vi "ENCOER_SUBVI.vi"(3 "Reset_Z":bool, 4 "Reset_Y":bool, 5 "Reset_X":bool) -> (0 "Position_Z":i16, 1 "Position_Y":i16, 2 "Position_X":i16)   [LabVIEW 2017]
uses:
  <vilib>/Platform/TimedLoop/XDataNode/timing_clust.ctl
  <vilib>/Platform/TimedLoop/XDataNode/nitl_modes.ctl
  <vilib>/Platform/TimedLoop/XDataNode/wakeup.ctl
  <vilib>/rvi/Emulation/niFpgaSctlEmulationGetInTimedLoop.vi
  <vilib>/rvi/Emulation/niFpgaEmulationReportErrorSimple.vi
  <vilib>/rvi/Emulation/niFpgaGetClockAttributes.vi
  <vilib>/rvi/Emulation/niFpgaCriticalErrorInLSC.vi
  <vilib>/rvi/eio/common/nirviEmuTemplateMethod_errors.vi
  <vilib>/Platform/TimedLoop/XDataNode/XDataNode.xnode
  <vilib>/eio/EIONode/EIONode.xnode
  <vilib>/Platform/TimedLoop/XDataNode/XDNodeRunTimeDep.lvlib
panel:
  # "Encoder Reader X Y Z"
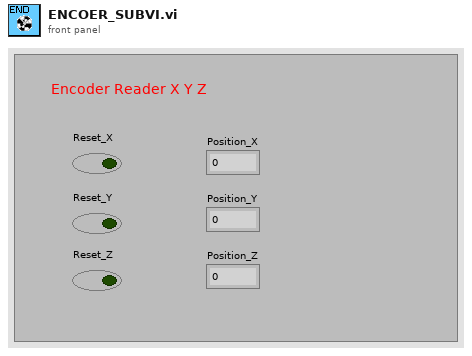
[diagram p1: front panel]
types:
  T1 = typedef "XDNodeRunTimeDep.lvlib/timing_clust.ctl" = cluster{"Expected End [f-1]":u64, "Actual End [f-1]":u64, "Finished Late? [f-1]":bool, "Expected End [i-1]":u64, "Actual End [i-1]":u64, "Finished Late? [i-1]":bool, "Expected Start [i]":u64, "Actual Start [i]":u64, "Expected Start [f]":u64, "Actual Start [f]":u64, "Source Name":string, "Structure Name":string, "Period":i64, "Deadline":i64, "Offset":i64, "Start":i64, "Priority":i32, "Timeout":i32, "Mode":T2, "Wakeup Reason":T3, "Error":errorcluster, "Source Type":string, "Secondary Source Type":string, "Global End Time":u64, "Global Start Time":u64, "Frame Duration":u64, "Iteration Duration":u64, "Assigned CPU":i32, "I/O Scan Engine Mode":u32}
  T2 = typedef "XDNodeRunTimeDep.lvlib/nitl_modes.ctl" = enum32{"No Change", "Process missed periods, maintain original phase", "Discard missed periods, maintain original phase", "Process missed periods, ignore original phase", "Discard missed periods, ignore original phase"}
  T3 = typedef "XDNodeRunTimeDep.lvlib/wakeup.ctl" = enum32{"Normal", "Aborted", "Asynchronous wakeup", "Timing source error", "Timed loop error", "Timeout"}
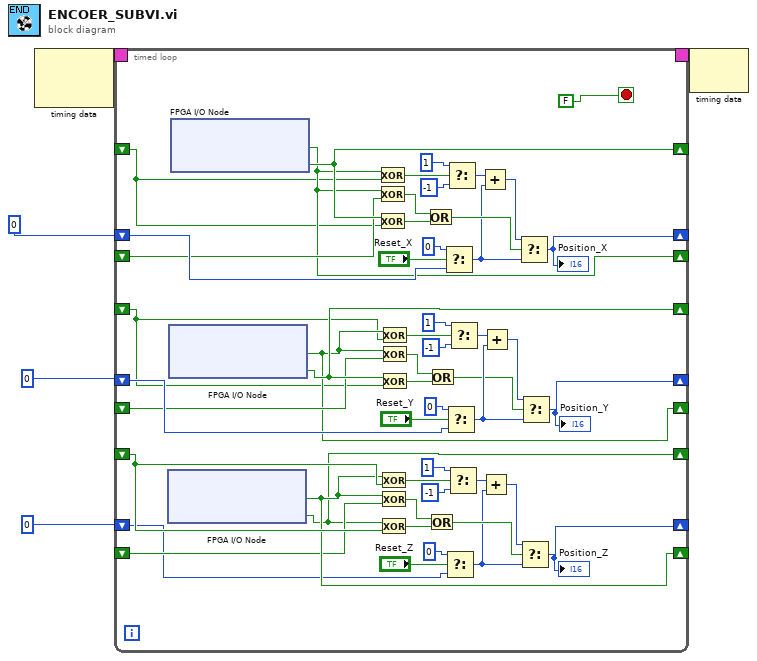
[diagram p0: block diagram]
diagram:
  n1 = node-c288() -> (w5:T1)  [unwired: 2 in]
  n2 = timed-loop {
    timing: w5 -> [_]
    timing-out: [_] -> w4
    shift-right: [w42] -> _
    shift-left: _ -> [w43]
    shift-right: [w44] -> _
    shift-left: _ -> [w41]
    shift-right: [w45] -> _
    shift-left: i16 0 ("f 3") -> [w49]
    shift-right: [w28] -> _
    shift-left: i16 0 ("f 2") -> [w29]
    shift-right: [w25] -> _
    shift-left: _ -> [w26]
    shift-right: [w27] -> _
    shift-left: _ -> [w24]
    shift-right: [w19] -> _
    shift-left: i16 0 ("f") -> [w18]
    shift-right: [w22] -> _
    shift-left: _ -> [w21]
    shift-right: [w20] -> _
    shift-left: _ -> [w23]
    stop <- FALSE stop-if-true
    n3 = xnode "FPGA I/O Node"() -> ("ConnectorA/DIO4"=w22:bool, "ConnectorA/DIO5"=w20:bool)  [unwired: 2 in, 2 out]
    n4 = xnode "FPGA I/O Node"() -> ("ConnectorA/DIO2"=w25:bool, "ConnectorA/DIO3"=w27:bool)  [unwired: 2 in, 2 out]
    n5 = xnode "FPGA I/O Node"() -> ("ConnectorA/DIO0"=w42:bool, "ConnectorA/DIO1"=w44:bool)  [unwired: 2 in, 2 out]
    n6 = Exclusive Or(1:w41, 2:w42) -> (0:w54:bool)
    n7 = Exclusive Or(1:w43, 2:w42) -> (0:w57:bool)
    n8 = Exclusive Or(1:w41, 2:w44) -> (0:w56:bool)
    n9 = Exclusive Or(1:w23, 2:w22) -> (0:w14:bool)
    n10 = Exclusive Or(1:w21, 2:w22) -> (0:w17:bool)
    n11 = Exclusive Or(1:w23, 2:w20) -> (0:w16:bool)
    n12 = Exclusive Or(1:w24, 2:w25) -> (0:w33:bool)
    n13 = Exclusive Or(1:w26, 2:w25) -> (0:w30:bool)
    n14 = Exclusive Or(1:w24, 2:w27) -> (0:w31:bool)
    n15 = Or(x=w57, y=w56) -> (x .or. y?=w48:bool)
    n16 = Or(x=w17, y=w16) -> (x .or. y?=w9:bool)
    n17 = Or(x=w30, y=w31) -> (x .or. y?=w38:bool)
    n18 = Select(t=i16 0 ("f"), s="Reset_X", f=w49) -> (s? t:f=w46:i16)
    n19 = Select(t=i16 0 ("f"), s="Reset_Z", f=w18) -> (s? t:f=w7:i16)
    n20 = Select(t=i16 0 ("f"), s="Reset_Y", f=w29) -> (s? t:f=w40:i16)
    n21 = Select(t=i16 1, s=w54, f=i16 -1) -> (s? t:f=w52:i16)
    n22 = Select(t=i16 1, s=w14, f=i16 -1) -> (s? t:f=w12:i16)
    n23 = Select(t=i16 1, s=w33, f=i16 -1) -> (s? t:f=w35:i16)
    n24 = Add(x=w52, y=w46) -> (x+y=w47:i16)
    n25 = Add(x=w12, y=w7) -> (x+y=w8:i16)
    n26 = Add(x=w35, y=w40) -> (x+y=w39:i16)
    n27 = Select(t=w47, s=w48, f=w46) -> (s? t:f=w45:i16)
    "Position_X" <- w45
    n28 = Select(t=w8, s=w9, f=w7) -> (s? t:f=w19:i16)
    "Position_Z" <- w19
    n29 = Select(t=w39, s=w38, f=w40) -> (s? t:f=w28:i16)
    "Position_Y" <- w28
  }
  n30 = node-c288(w4) -> ()  [unwired: 1 out]
